vi "Test Stock Table - Animate - 01.vi"(8 "error in (no error)":errorcluster, 11 "TestCase in":refnum<class "TestCase.lvclass">) -> (0 "error out":errorcluster, 3 "TestCase out":refnum<class "TestCase.lvclass">)   [LabVIEW 2011, in "test.lvclass"]
uses:
  test.lvclass
  <vilib>/addons/_JKI Toolkits/VI Tester/TestCase.llb/TestCase.lvclass
panel:
  in  "Table":string[][](table)
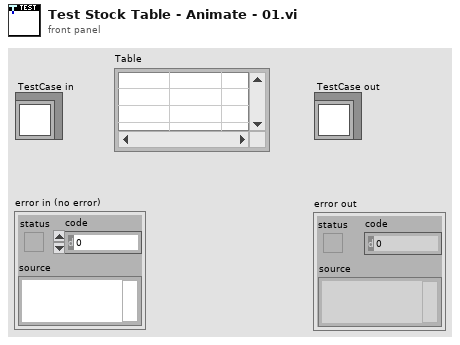
[diagram p1: front panel]
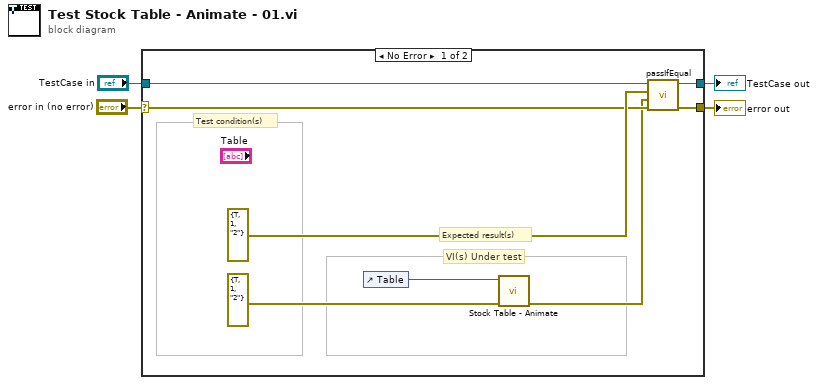
[diagram p0: block diagram]
diagram:
  n1 = case shown="No Error" "error in (no error)" {
    selector: "error in (no error)" -> [w10 w13]
    tunnel: "TestCase in" -> [w11 w14]
    tunnel: [w6 w14] -> w3
    tunnel: [w5 w13] -> w2
    frame No Error {
      # "Expected result(s)"
      # "Test condition(s)"
      # "VI(s) Under test"
      n2 = control-ref of="Table"() -> (w9:refnum<vi>)
      n3 = call "Stock Table - Animate.vi"("error in"=errorcluster {"status"=TRUE, "code"=1, "source"="2"} ("error in (no error)"), "Table Reference"=w9) -> ("error out"=w7:errorcluster)  [unwired: 9 in]
      n4 = call-dynamic "passIfEqual.vi"("error in (no error)"=w10, "y"=w7, "x"=errorcluster {"status"=TRUE, "code"=1, "source"="2"} ("error in (no error)"), "TestCase in"=w11) -> ("error out"=w5:errorcluster, "TestCase out"=w6:refnum<class "TestCase.lvclass">)  [unwired: 6 in]
    }
    frame Error {
    }
  }
  "TestCase out" <- w3
  "error out" <- w2
